vi "CreateIterator.vi"(8 "error in (no error)":errorcluster, 11 "BrowerComposite in":refnum<class "BrowerComposite.lvclass">) -> (0 "error out":errorcluster, 2 "Iterator":refnum<class "Iterator.lvclass">, 3 "BrowerComposite out":refnum<class "BrowerComposite.lvclass">)   [LabVIEW 2015, in "BrowerComposite.lvclass"]
uses:
  BrowerComposite.lvclass
  Iterator/ArrayIterator/ArrayIterator.lvclass
  Association/iRobotDebugSystem/Browers/Iterator/CompositeIterator/CompositeIterator.lvclass
  Association/iRobotDebugSystem/Browers/Iterator/Interface Iterator/Iterator.lvclass
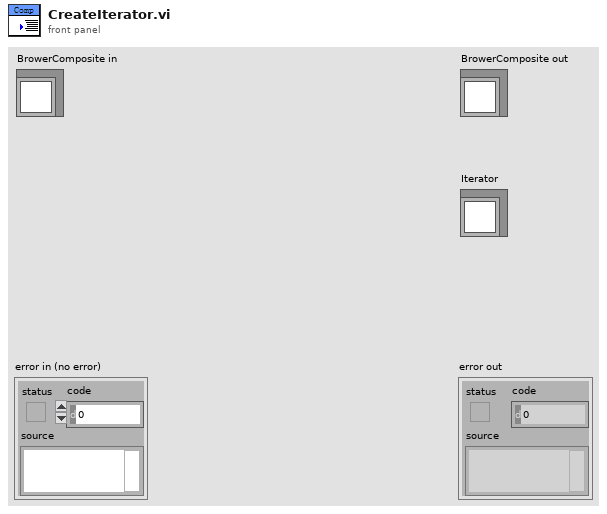
[diagram p1: front panel]
types:
  T1 = typedef "BrowerComposite.lvclass/ObjectAttributes.ctl" = cluster{"BrowerComponents":refnum<class "BrowerComponent.lvclass">[], "BrowerComponentIDs":string[]}
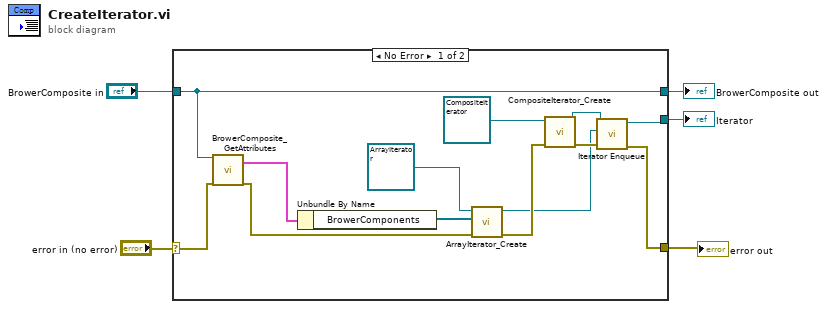
[diagram p0: block diagram]
diagram:
  n1 = case shown="No Error" "error in (no error)" {
    selector: "error in (no error)" -> [w17 w19]
    tunnel: "BrowerComposite in" -> [w18 w20]
    tunnel: [w18 w20] -> w4
    tunnel: [w7 w19] -> w3
    tunnel: [w6 _] -> w1
    frame No Error {
      n2 = call "BrowerComposite_GetAttributes.vi"("reference in"=w18, "error in (no error)"=w17) -> ("Data"=w16:T1, "error out"=w13:errorcluster)  [unwired: 14 in, 2 out]
      n3 = Unbundle By Name(w16) -> ("BrowerComponents"=w15:refnum<class "BrowerComponent.lvclass">[])
      n4 = call "ArrayIterator_Create.vi"("error in (no error)"=w13, "BrowerComponents"=w15, "reference in"=refnum<class "ArrayIterator.lvclass"> refnum) -> ("error out"=w11:errorcluster, "reference out"=w8:refnum<class "ArrayIterator.lvclass">)  [unwired: 7 in]
      n5 = call "CompositeIterator_Create.vi"("error in (no error)"=w11, "reference in"=refnum<class "CompositeIterator.lvclass"> refnum) -> ("error out"=w9:errorcluster, "reference out"=w10:refnum<class "CompositeIterator.lvclass">)  [unwired: 8 in]
      n6 = call-dynamic "Iterator Enqueue.vi"("error in (no error)"=w9, "Iterator"=w8, "CompositeIterator in"=w10) -> ("error out"=w7:errorcluster, "CompositeIterator out"=w6:refnum<class "CompositeIterator.lvclass">)  [unwired: 7 in]
    }
    frame Error {
    }
  }
  "error out" <- w3
  "BrowerComposite out" <- w4
  "Iterator" <- w1
